vi "MasterAquisitionFile_2P_V2.vi"() -> ()   [LabVIEW 2020]
uses:
  <vilib>/userDefined/High Color/IMAQdx.ctl
  <vilib>/vision/driver/IMAQdx.llb/IMAQdx Camera Control Mode.ctl
  <vilib>/vision/driver/IMAQdx.llb/IMAQdx Acquisition Mode.ctl
  <vilib>/vision/driver/IMAQdx.llb/IMAQdx Buffer Number Mode.ctl
  <vilib>/DAQmx/write.llb/DAQmx Write (Digital 1D Wfm NChan NSamp).vi
  <vilib>/DAQmx/read.llb/DAQmx Read (Digital 1D Bool 1Chan 1Samp).vi
  <vilib>/DAQmx/read.llb/DAQmx Read (Analog 1D Wfm NChan NSamp).vi
  <vilib>/Waveform/DWDTOps.llb/DWDT Digital to Boolean Array.vi
  <vilib>/DAQmx/create/channels.llb/DAQmx Create Channel (DO-Digital Output).vi
  <vilib>/DAQmx/configure/timing.llb/DAQmx Timing (Sample Clock).vi
  <vilib>/Waveform/DWDTOps.llb/DWDT Uncompress Digital.vi
  <vilib>/DAQmx/miscellaneous.llb/DAQmx Fill In Error Info.vi
  <vilib>/DAQmx/create/channels.llb/DAQmx Create Channel (DI-Digital Input).vi
  <vilib>/DAQmx/create/channels.llb/DAQmx Create Channel (AI-Voltage-Basic).vi
  <vilib>/DAQmx/configure/trigger.llb/DAQmx Start Trigger (Digital Edge).vi
  <vilib>/DAQmx/create/channels.llb/DAQmx Create Channel (CO-Pulse Generation-Frequency).vi
  <vilib>/DAQmx/configure/timing.llb/DAQmx Timing (Implicit).vi
  <vilib>/vision/driver/NI_Vision_Acquisition_Software.lvlib
  <resource>/objmgr/imaqdx.rc
  <resource>/objmgr/daqmx.rc
panel:
  out "Auditory":bool
  out "RPad":bool
  out "LPad":bool
  in  "Sol Stim Parameters":cluster{"Fs":dbl, "Samples":dbl}
  in  "LED Stim Parameters":cluster{"Fs":dbl, "Samples":dbl}
  in  "Generate Stimuli":bool=TRUE
  in  "Sol Duty Cycle (%)":dbl=10.0
  in  "Sol Freq":dbl=1.0
  in  "Sol Dur (s)":dbl=1.0
  in  "LED Duty Cycle (%)":dbl=10.0
  in  "LED Freq":dbl=10.0
  in  "LED Dur (s)":dbl=2.0
  out "Stimulus Order":digitalwaveform[](graph)=[{"t0"=timestamp(0 s since 1904-01-01), "dt"=5e-05, "Y"={"transitions"=[], "data"=array18000000x1[18000000 elements]}}, {"t0"=timestamp(0 s since 1904-01-01), "dt"=5e-05, "Y"={"transitions"=[], "data"=array18000000x1[18000000 elements]}}, {"t0"=timestamp(0 s since 1904-01-01), "dt"=5e-05, "Y"={"transitions"=[], "data"=array18000000x1[18000000 elements]}}, {"t0"=timestamp(0 s since 1904-01-01), "dt"=5e-05, "Y"={"transitions"=[], "data"=array18000000x1[18000000 elements]}}]
  out "Solenoid Stim":digitalwaveform(graph)={"t0"=timestamp(0 s since 1904-01-01), "dt"=5e-05, "Y"={"transitions"=[], "data"=array20000x1[20000 elements]}}
  in  "Trial Offset (s)":dbl=15.0
  in  "Interstim (s)":dbl=30.0
  in  "Right Pad":dbl=1.0
  in  "Left Pad":dbl=1.0
  in  "Auditory":dbl=1.0
  in  "LED":dbl
  out "?":T1(plugin-control)
  out "Web Cam Fs 2":dbl(knob) scale=0.0..200.0
  out "MScan Cam":bool
  out "?":T1(plugin-control)
  in  "stop":bool
  out "?":T1(plugin-control)
  out "Web Cam Fs":dbl(knob) scale=0.0..200.0
  out "Behav Cam":bool
  out "Complete":bool
  out "Whisk Cam":bool
  out "Analog":bool
  out "MScan Trig":bool
  out "?":bool[](array[boolean])=[TRUE]
  out "Hexadecimal Data":u32=1 format="%x"
  out "Time Elapsed (Min)":cluster{dbl, dbl}(slide)={16.0, 0.028422350000000002} scale=0.0..16.0 scale format="%#_2g"
  out "Whisker Camera":bool
  out "Analog Data":bool
  out "Analog Samples":i32
  in  "Analog Channel\n Labels":string[](array[string])=["forceSensor", "AudSol", "LPadSol", "RPadSol", "", "", "", ""]
  in  "?":cluster{"Analog Fs":u16}={"Analog Fs"=20000} {"Analog Fs" format="%0.0f"}
  in  "?":cluster{"WhiskerCam Fs":u16}={"WhiskerCam Fs"=150}
  out "Notes Size":i32=7
  out "Notes Reversed":string[](array[string])=["Experimenter", "Animal ID", "Isoflurane time", "Amplifier Gain", "Session ID", "Hemisphere", "Solenoid PSI"]
  out "Notes Array":string[](array[string])=["Solenoid PSI", "Hemisphere", "Session ID", "Amplifier Gain", "Isoflurane time", "Animal ID", "Experimenter"]
  in  "Notes:":T2={"Experimenter"="Kevin\n", "Animal ID"="T201", "Isoflurane time"="1110", "Amplifier Gain"="10000", "Session ID"="Imaging Session Three", "Hemisphere"="RH", "Solenoid PSI"="10"}
  in  "Target Path":path=path "C:/Users/klt8/Documents/T201/Imaging Session 3 - 7 Apr. 2021" caption="Final Saved File Location"
  out "Dropped":u32(slide) caption="Whisk Cam" scale=0.0..150.0
  out "Current File Name":string="190611_17_21_53"
  in  "Time (min)":dbl(knob)=16.0 min=0.5 max=20.0 step=0.5 scale=0.0..20.0 scale format="%#_3g"
  in  "Temp Path":path=path "C:/Users/klt8/Documents/LabVIEW Temp Files" caption="Temporary File Path"
  out "Last Whisk Buffer":u32=251
  out "Whisk Cam Fs":dbl(knob) scale=0.0..200.0 scale format="%#1_6g"
  # "Notes"
  # "Dropped Frames"
  # "LPAD"
  # "RPAD"
  # "AUD"
  # "AnalogFs"
  # "WhiskFs"
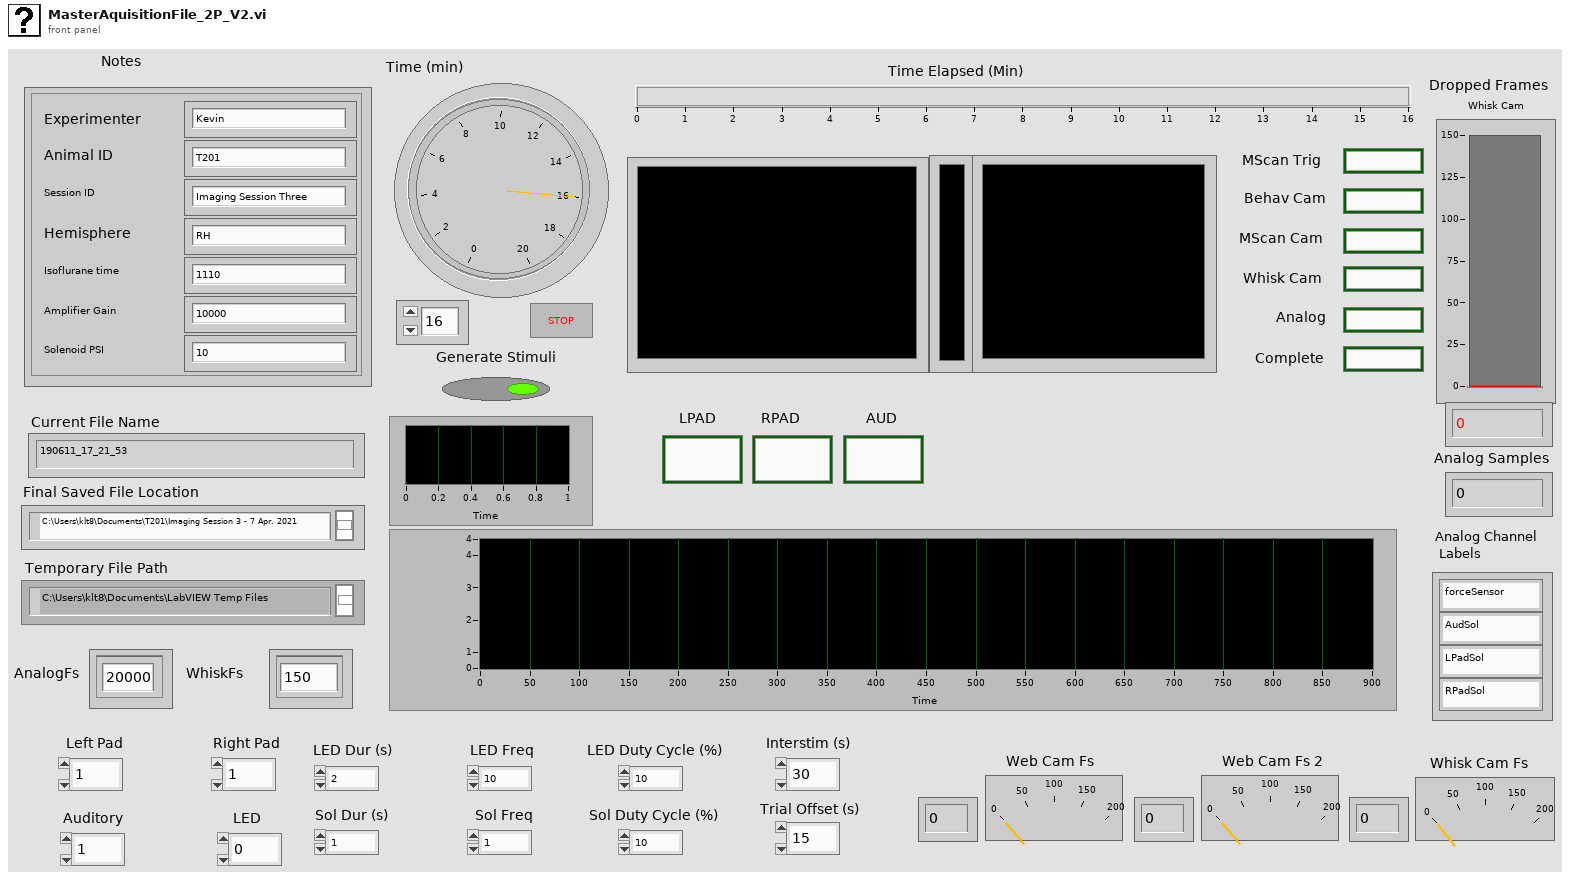
[diagram p1: front panel]
types:
  T1 = typedef "IMAQ Image.ctl" = refnum<image>
  T2 = cluster{"Experimenter":string, "Animal ID":string, "Isoflurane time":string, "Amplifier Gain":string, "Session ID":string, "Hemisphere":string, "Solenoid PSI":string}
  T3 = typedef "IMAQdx.ctl" = refnum<k21>
  T4 = typedef "NI_Vision_Acquisition_Software.lvlib/IMAQdx Camera Control Mode.ctl" = enum32{"Controller", "Listener"}
  T5 = enum16{"open", "open or create", "create or replace", "create", "open (read-only)"}
  T6 = enum16{"open", "replace", "create", "open or create", "replace or create", "replace or create with confirmation"}
  T7 = typedef "NI_Vision_Acquisition_Software.lvlib/IMAQdx Acquisition Mode.ctl" = enum32{"One Shot", "Continuous"}
  T8 = enum16{"big-endian, network order", "native, host order", "little-endian"}
  T9 = typedef "NI_Vision_Acquisition_Software.lvlib/IMAQdx Buffer Number Mode.ctl" = enum32{"Next", "Last", "Buffer Number", "Every", "Last New"}
  T10 = typedef "Image Type" = u32
  T11 = typedef "IMAQ AVI2 Refnum.ctl" = refnum<k20>
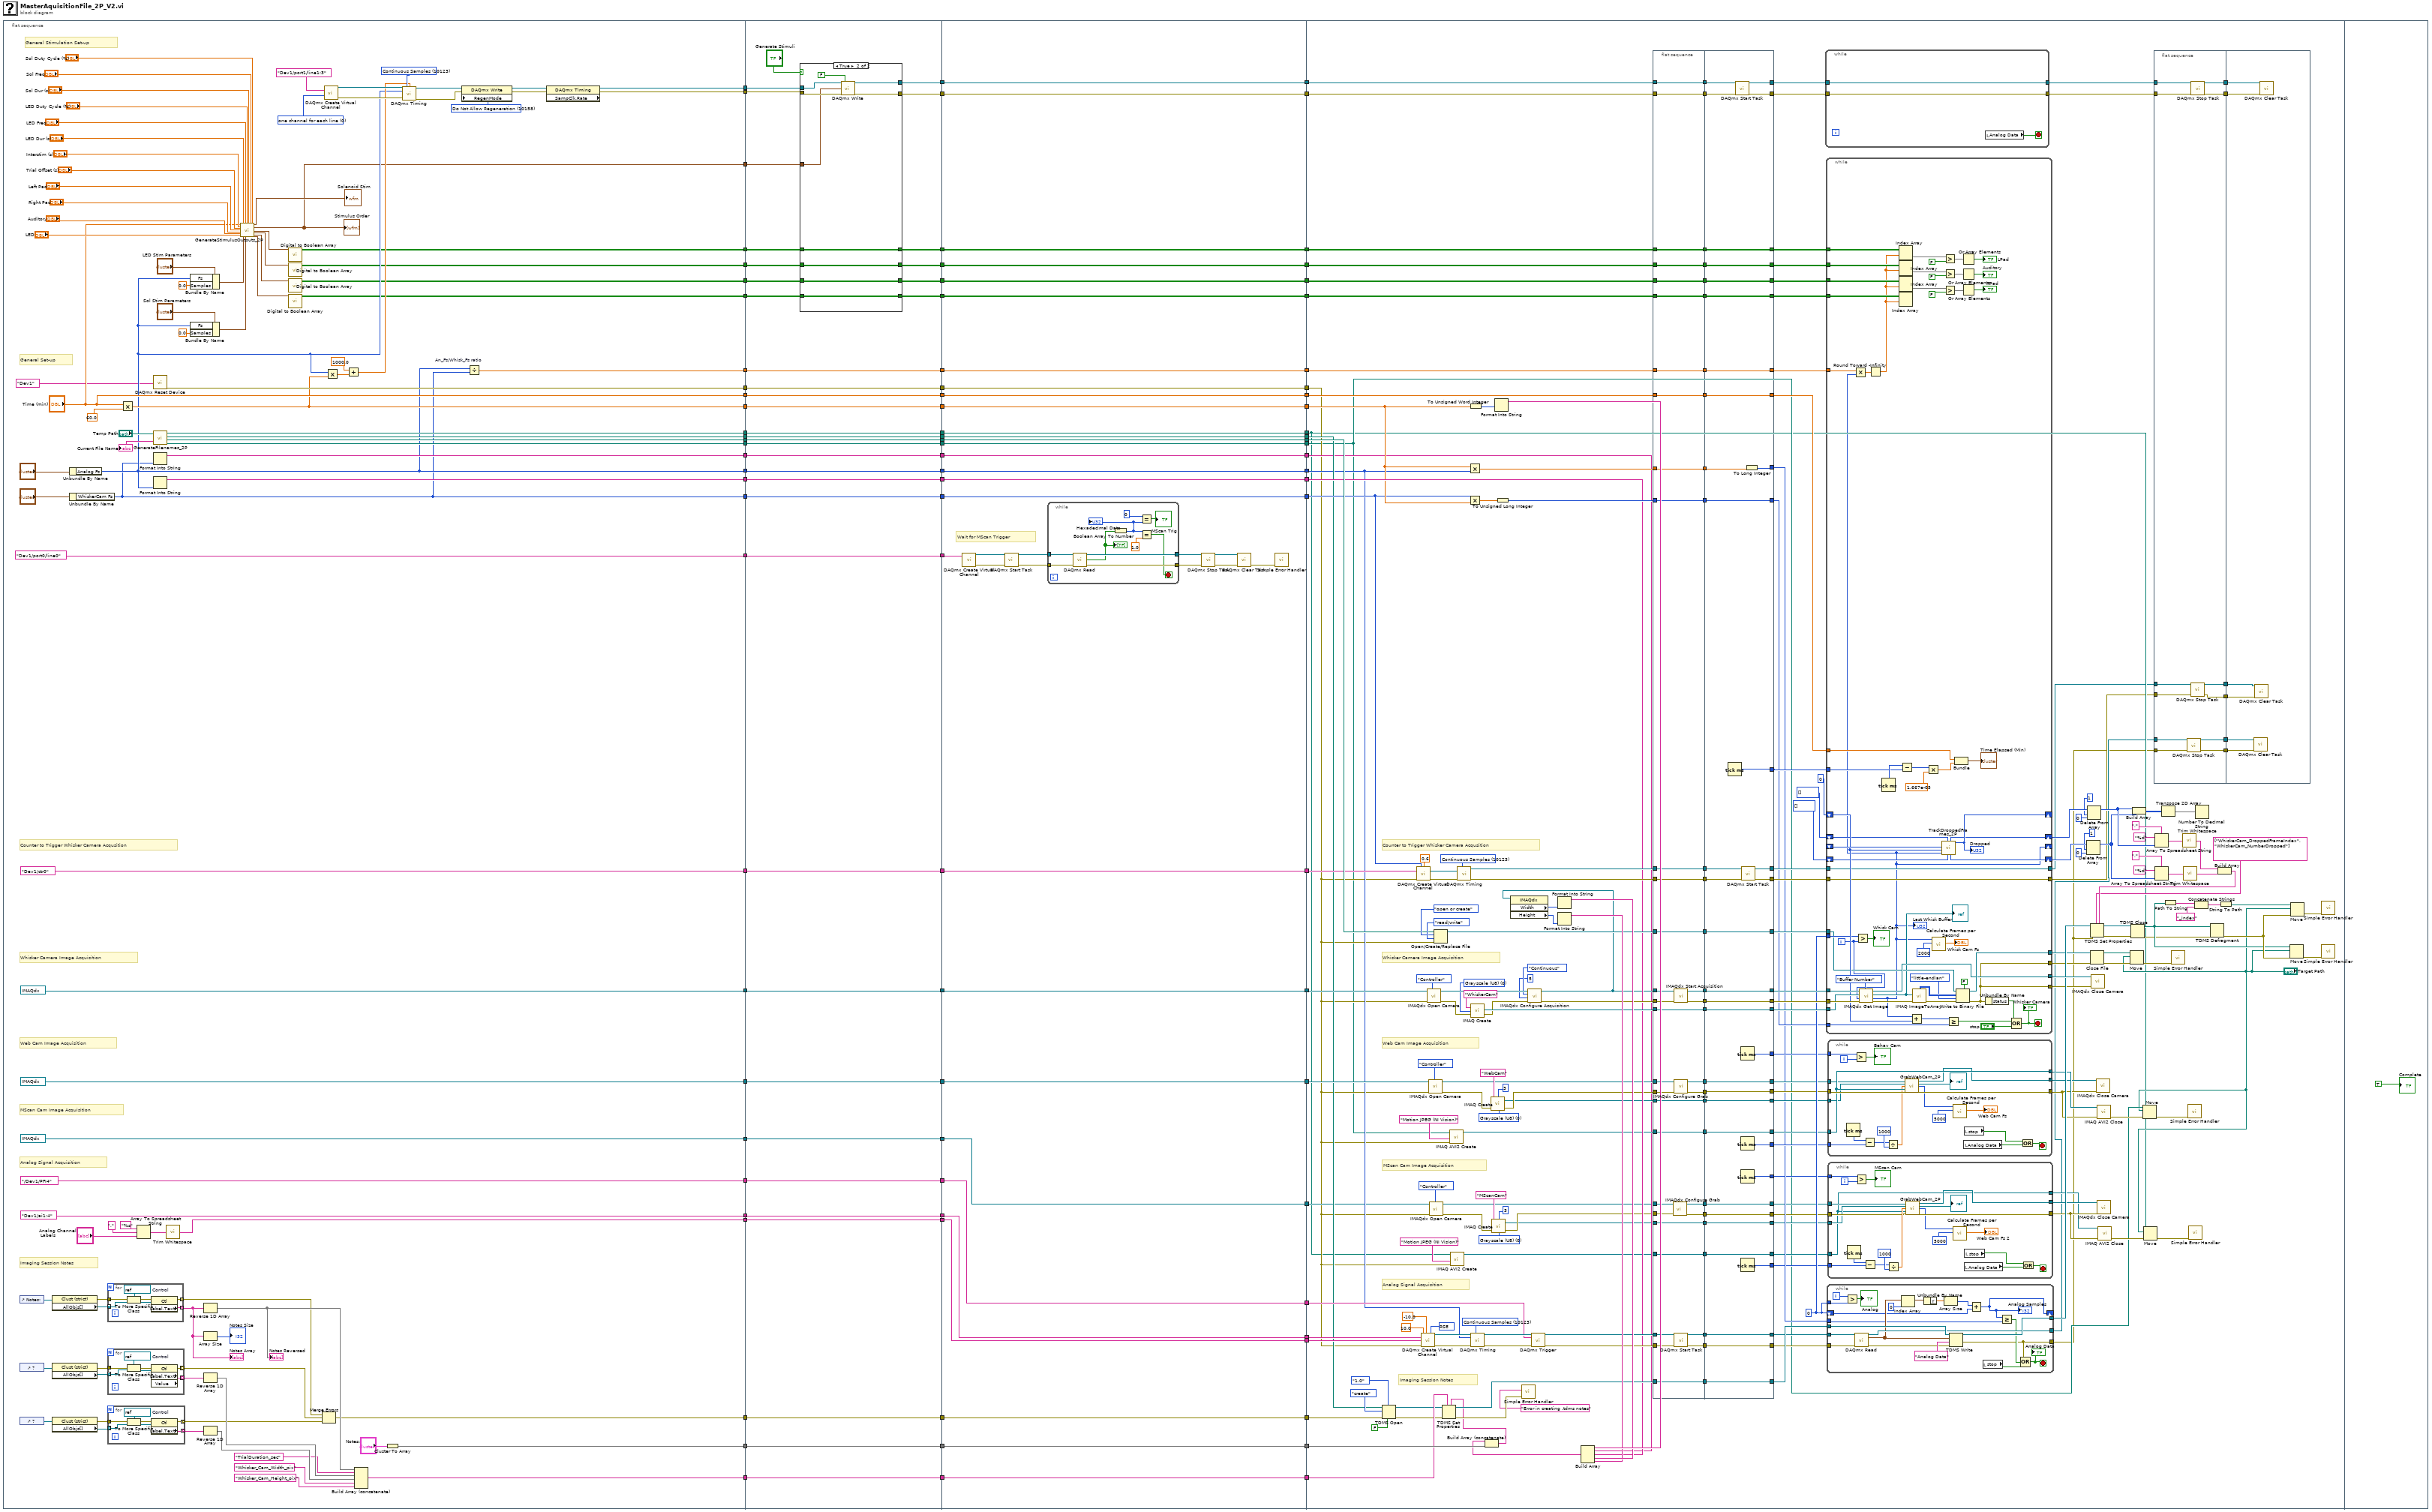
[diagram p0: block diagram]
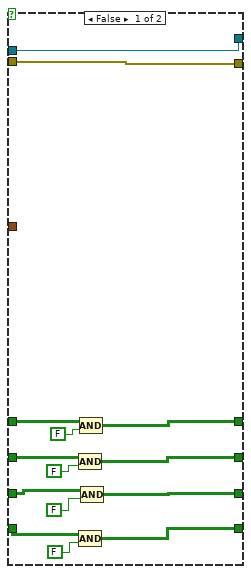
[diagram p2: hidden frame]
diagram:
  n1 = flat-sequence {
    tunnel: [tag "/Dev1/PFI4" ("Whisk Cam Trigger")] -> w59
    tunnel: [w109] -> w57
    tunnel: ["Time (min)"] -> w55
    tunnel: [w156] -> w53
    tunnel: [w155] -> w51
    tunnel: [w107] -> w49
    tunnel: [w106] -> w47
    tunnel: [w154] -> w45
    tunnel: [tag "Dev1/ctr0" ("Whisk Cam Counter")] -> w43
    tunnel: [w153] -> w41
    tunnel: [tag "Dev1/ai1:4" ("Analog Input Channels")] -> w39
    tunnel: [T3 "cam1" ("Whisker Cam ID")] -> w37
    tunnel: [w152] -> w35
    tunnel: [w150] -> w33
    tunnel: [w151] -> w31
    tunnel: [T3 "cam2" ("WebCam ID")] -> w29
    tunnel: [tag "Dev1/port0/line0" ("MScan Trigger")] -> w27
    tunnel: [w147] -> w25
    tunnel: [w146] -> w23
    tunnel: [w145] -> w21
    tunnel: [T3 "cam7" ("WebCam ID 2")] -> w19
    tunnel: [w144] -> w17
    tunnel: [w105] -> w9
    tunnel: [w94] -> w7
    tunnel: [w93] -> w6
    tunnel: [w92] -> w5
    tunnel: [w91] -> w4
    tunnel: [w90] -> w3
    tunnel: [w89] -> w2
    tunnel: [w88] -> w1
    tunnel: w59 -> [w244]
    tunnel: [w244] -> w58
    tunnel: w57 -> [w243]
    tunnel: [w243] -> w56
    tunnel: w55 -> [w242]
    tunnel: [w242] -> w54
    tunnel: w53 -> [w241]
    tunnel: [w241] -> w52
    tunnel: w51 -> [w240]
    tunnel: [w240] -> w50
    tunnel: w49 -> [w239]
    tunnel: [w239] -> w48
    tunnel: w47 -> [w238]
    tunnel: [w238] -> w46
    tunnel: w45 -> [w237]
    tunnel: [w237] -> w44
    tunnel: w43 -> [w236]
    tunnel: [w236] -> w42
    tunnel: w41 -> [w235]
    tunnel: [w235] -> w40
    tunnel: w39 -> [w234]
    tunnel: [w234] -> w38
    tunnel: w37 -> [w233]
    tunnel: [w233] -> w36
    tunnel: w35 -> [w232]
    tunnel: [w232] -> w34
    tunnel: w33 -> [w231]
    tunnel: [w231] -> w32
    tunnel: w31 -> [w230]
    tunnel: [w230] -> w30
    tunnel: w29 -> [w229]
    tunnel: [w229] -> w28
    tunnel: w27 -> [w228]
    tunnel: [w228] -> w26
    tunnel: w25 -> [w227]
    tunnel: [w227] -> w24
    tunnel: w23 -> [w226]
    tunnel: [w226] -> w22
    tunnel: w21 -> [w225]
    tunnel: [w225] -> w20
    tunnel: w19 -> [w224]
    tunnel: [w224] -> w18
    tunnel: w17 -> [w223]
    tunnel: [w223] -> w16
    tunnel: [w214] -> w15
    tunnel: [w213] -> w14
    tunnel: [w212] -> w13
    tunnel: [w211] -> w12
    tunnel: [w210] -> w11
    tunnel: [w209] -> w10
    tunnel: w9 -> [w222]
    tunnel: [w222] -> w8
    tunnel: w7 -> [w221]
    tunnel: w6 -> [w220]
    tunnel: w5 -> [w219]
    tunnel: w4 -> [w218]
    tunnel: w3 -> [w217]
    tunnel: w2 -> [w216]
    tunnel: w1 -> [w215]
    tunnel: [w283] -> w87
    tunnel: [w295] -> w86
    tunnel: [w296] -> w85
    tunnel: [w297] -> w84
    tunnel: [w298] -> w83
    tunnel: [w285] -> w82
    tunnel: [w299] -> w81
    tunnel: [w284] -> w80
    tunnel: [w300] -> w79
    tunnel: [w301] -> w78
    tunnel: [w302] -> w77
    tunnel: [w303] -> w76
    tunnel: [w304] -> w75
    tunnel: [w305] -> w74
    tunnel: [w306] -> w73
    tunnel: w58 -> [w306]
    tunnel: w56 -> [w305]
    tunnel: w54 -> [w304]
    tunnel: w52 -> [w303]
    tunnel: w50 -> [w302]
    tunnel: w48 -> [w301]
    tunnel: w46 -> [w300]
    tunnel: w44 -> [w284]
    tunnel: w42 -> [w299]
    tunnel: w40 -> [w285]
    tunnel: w38 -> [w298]
    tunnel: w36 -> [w297]
    tunnel: w34 -> [w296]
    tunnel: w32 -> [w295]
    tunnel: w30 -> [w283]
    tunnel: [w281] -> w72
    tunnel: w28 -> [w281]
    tunnel: w26 -> [w282]
    tunnel: w24 -> [w280]
    tunnel: [w280] -> w71
    tunnel: w22 -> [w279]
    tunnel: w20 -> [w278]
    tunnel: [w279] -> w70
    tunnel: [w278] -> w69
    tunnel: w18 -> [w277]
    tunnel: [w277] -> w68
    tunnel: w16 -> [w276]
    tunnel: [w276] -> w67
    tunnel: [w275] -> w66
    tunnel: w15 -> [w275]
    tunnel: [w274] -> w65
    tunnel: w14 -> [w274]
    tunnel: [w273] -> w64
    tunnel: w13 -> [w273]
    tunnel: [w272] -> w63
    tunnel: w12 -> [w272]
    tunnel: [w271] -> w62
    tunnel: w11 -> [w271]
    tunnel: w10 -> [w270]
    tunnel: [w270] -> w61
    tunnel: [w269] -> w60
    tunnel: w8 -> [w269]
    tunnel: w87 -> [w429]
    tunnel: w86 -> [w439]
    tunnel: w85 -> [w373]
    tunnel: w84 -> [w438]
    tunnel: w83 -> [w437]
    tunnel: w82 -> [w436]
    tunnel: w81 -> [w435]
    tunnel: w80 -> [w434]
    tunnel: w79 -> [w398]
    tunnel: w78 -> [w388]
    tunnel: w77 -> [w433]
    tunnel: w76 -> [w387]
    tunnel: w75 -> [w426]
    tunnel: w74 -> [w432]
    tunnel: w73 -> [w431]
    tunnel: w72 -> [w417]
    tunnel: w71 -> [w352]
    tunnel: w70 -> [w394]
    tunnel: w69 -> [w392]
    tunnel: w68 -> [w375]
    tunnel: w67 -> [w350]
    tunnel: w66 -> [w320]
    tunnel: w65 -> [w318]
    tunnel: w64 -> [w324]
    tunnel: w63 -> [w323]
    tunnel: w62 -> [w322]
    tunnel: w61 -> [w321]
    tunnel: w60 -> [w340]
    frame #0 {
      w124 = 10158 items=["Allow Regeneration"=10097, "Do Not Allow Regeneration"=10158] ("RegenMode")
      w125 = 10123 items=["Finite Samples"=10178, "Continuous Samples"=10123, "Hardware Timed Single Point"=12522] ("sample mode")
      w128 = 0 items=["one channel for each line", "one channel for all lines"] ("line grouping")
      # "General Stimulation Set-up"
      # "MScan Cam Image Acquisition"
      # "General Set-up"
      # "Whisker Camera Image Acquisition"
      # "Imaging Session Notes"
      # "Counter to Trigger Whisker Camera Acqusition"
      # "Web Cam Image Acquisition"
      # "Analog Signal Acquisition"
      n2 = control-ref of="Notes:"() -> (w172:refnum<vi>)
      n3 = control-ref of="?"() -> (w170:refnum<vi>)
      n4 = control-ref of="?"() -> (w163:refnum<vi>)
      n5 = property class="Clust (strict)"(reference=w172) -> (error out=w171:errorcluster, "AllObjs[]"=w173:refnum<vi>[])  [unwired: 1 in, 1 out]
      n6 = property class="Clust (strict)"(reference=w170) -> (error out=w168:errorcluster, "AllObjs[]"=w169:refnum<vi>[])  [unwired: 1 in, 1 out]
      n7 = property class="Clust (strict)"(reference=w163) -> (error out=w164:errorcluster, "AllObjs[]"=w166:refnum<vi>[])  [unwired: 1 in, 1 out]
      n8 = Unbundle By Name("?") -> ("Analog Fs"=w107:u16)
      n9 = Unbundle By Name("?") -> ("WhiskerCam Fs"=w106:u16)
      n10 = for {
        tunnel: [w191] -> w178 mode=indexing
        tunnel: w173 -> [w190] mode=indexing
        tunnel: w171 -> [w189]
        tunnel: [w187] -> w177 mode=indexing
        w192 = refnum<vi> refnum  # Control
        n11 = To More Specific Class(target class=w192, reference=w190, error in=w189) -> (specific class reference=w193:refnum<vi>, error out=w188:errorcluster)
        n12 = property class="Ctl"(reference=w193, error in=w188) -> (error out=w187:errorcluster, "Label.Text"=w191:string)  [unwired: 1 out]
      }
      "Notes Array" <- w178
      n13 = for {
        tunnel: [w198] -> w167 mode=indexing
        tunnel: w169 -> [w197] mode=indexing
        tunnel: w168 -> [w196]
        tunnel: [w194] -> w176 mode=indexing
        w199 = refnum<vi> refnum  # Control
        n14 = To More Specific Class(target class=w199, reference=w197, error in=w196) -> (specific class reference=w200:refnum<vi>, error out=w195:errorcluster)
        n15 = property class="Ctl" props=["Label", "Text", "Value"](reference=w200, error in=w195) -> (error out=w194:errorcluster, "Label.Text"=w198:string)  [unwired: 2 out]
      }
      n16 = for {
        tunnel: [w205] -> w165 mode=indexing
        tunnel: w166 -> [w204] mode=indexing
        tunnel: w164 -> [w203]
        tunnel: [w201] -> w175 mode=indexing
        w206 = refnum<vi> refnum  # Control
        n17 = To More Specific Class(target class=w206, reference=w204, error in=w203) -> (specific class reference=w207:refnum<vi>, error out=w202:errorcluster)
        n18 = property class="Ctl"(reference=w207, error in=w202) -> (error out=w201:errorcluster, "Label.Text"=w205:string)  [unwired: 1 out]
      }
      n19 = Multiply(x="Time (min)", y=60.0) -> (x*y=w109:dbl)
      n20 = Array To Spreadsheet String(delimiter (Tab)=",", array="Analog Channel\n Labels", 3:"%s" ("format string")) -> (spreadsheet string=w180:string)
      n21 = call <vilib>:"DAQmx Reset Device.vi"("device in"=tag "Dev1" ("NI Board")) -> ("error out"=w152:errorcluster)  [unwired: 14 in]
      n22 = call "GenerateFilenames_2P.vi"("path"="Temp Path") -> ("WebCam Path"=w147:path, "Basler Path"=w150:path, "TDMS Path"=w145:path, "MScan Path"=w144:path, "Analog file name"=→"Current File Name":string)  [unwired: 2 in]
      n23 = Format Into String(w106) -> (resulting string=w156:string)  [unwired: 3 in, 1 out]
      n24 = Format Into String(w107) -> (resulting string=w155:string)  [unwired: 3 in, 1 out]
      n25 = call <vilib>:"Trim Whitespace.vi"("string"=w180) -> ("trimmed string"=w153:string)  [unwired: 1 in]
      n26 = Bundle By Name(cluster="LED Stim Parameters", "Fs"=w107, "Samples"=0.0) -> (w114:cluster{"Fs":dbl, "Samples":dbl})
      n27 = Bundle By Name(cluster="Sol Stim Parameters", "Fs"=w107, "Samples"=0.0) -> (w113:cluster{"Fs":dbl, "Samples":dbl})
      n28 = Reverse 1D Array(array=w178) -> (reversed array=w179:string[])
      "Notes Reversed" <- w179
      n29 = Array Size(array=w178) -> (size(s)=→"Notes Size":i32)
      n30 = Reverse 1D Array(array=w167) -> (reversed array=w185:string[])
      n31 = Reverse 1D Array(array=w165) -> (reversed array=w186:string[])
      n32 = call "GenerateStimulusOutputs_2P.vi"("Trial duration (min)"="Time (min)", "Rest duration(s)"="Interstim (s)", "trial offset (s)"="Trial Offset (s)", "Left Pad"="Left Pad", "Right Pad"="Right Pad", "Auditory"="Auditory", "LED"="LED", "LED Stim Duration (s)"="LED Dur (s)", "LED Stim Parameters"=w114, "LED Frequency"="LED Freq", "Sol Stim Parameters"=w113, "LED duty cycle (%)"="LED Duty Cycle (%)", "Sol Stim Duration (s)"="Sol Dur (s)", "Sol Frequency"="Sol Freq", "Sol Duty Cycle (%)"="Sol Duty Cycle (%)") -> ("Solenoid Stim Waveforms"=→"Solenoid Stim":digitalwaveform, "Stimulus Digital Outputs"=w90:digitalwaveform[], "Left Pad Out"=w103:digitalwaveform, "Auditory Out"=w130:digitalwaveform, "Right Pad Out"=w129:digitalwaveform, "LED Out"=w108:digitalwaveform)  [unwired: 7 in]
      "Stimulus Order" <- w90
      n33 = call-poly <vilib>:"Digital to Boolean Array.vi"("digital waveform"=w103) -> ("boolean array"=w89:bool[][])  [unwired: 9 in, 1 out]
      n34 = call-poly <vilib>:"Digital to Boolean Array.vi"("digital waveform"=w130) -> ("boolean array"=w92:bool[][])  [unwired: 9 in, 1 out]
      n35 = call-poly <vilib>:"Digital to Boolean Array.vi"("digital waveform"=w129) -> ("boolean array"=w91:bool[][])  [unwired: 9 in, 1 out]
      n36 = call-poly <vilib>:"Digital to Boolean Array.vi"("digital waveform"=w108) -> ("boolean array"=w88:bool[][])  [unwired: 9 in, 1 out]
      n37 = Merge Errors(w177, w176, w175) -> (w146:errorcluster)
      n38 = call-poly <vilib>:"DAQmx Create Virtual Channel.vi"("lines"=tag "Dev1/port1/line1:3", "line grouping"=w128) -> ("task out"=w127:refnum<k21>, "error out"=w126:errorcluster)  [unwired: 12 in]
      n39 = Multiply(x=w107, y=w109) -> (x*y=w112:dbl)
      n40 = Add(x=1000.0, y=w112) -> (x+y=w110:dbl)
      n41 = Build Array (concatenate)(w179, "TrialDuration_sec", w185, w186, "Whisker_Cam_Width_pix", "Whisker_Cam_Height_pix") -> (w151:string[])
      n42 = Cluster To Array(cluster="Notes:") -> (array=w154:string[])
      n43 = call-poly <vilib>:"DAQmx Timing.vi"("task/channels in"=w127, "sample mode"=w125, "samples per channel"=w110, "rate"=w107, "error in"=w126) -> ("task out"=w121:refnum<k21>, "error out"=w120:errorcluster)  [unwired: 9 in]
      n44 = property class="DAQmx Write"(reference=w121, error in=w120, "RegenMode"=w124) -> (reference out=w122:refnum<k21>, error out=w123:errorcluster)
      n45 = Divide "An_Fs/Whisk_Fs ratio"(x=w107, y=w106) -> (x/y=w105:dbl)
      n46 = property class="DAQmx Timing" props=["SampClk.Rate"](reference=w122, error in=w123) -> (reference out=w94:refnum<k21>, error out=w93:errorcluster)  [unwired: 1 out]
    }
    frame #1 {
      n47 = case shown="True" "Generate Stimuli" {
        tunnel: w221 -> [w258 w268]
        tunnel: w220 -> [w257 w267]
        tunnel: [w258 w266] -> w214
        tunnel: [w257 w265] -> w213
        tunnel: w219 -> [w253 w264]
        tunnel: w218 -> [w254 w263]
        tunnel: [w247 w261] -> w212
        tunnel: [w256 w264] -> w211
        tunnel: [w255 w263] -> w210
        tunnel: [w246 w260] -> w209
        tunnel: w217 -> [_ w262]
        tunnel: w216 -> [w248 w261]
        tunnel: w215 -> [w245 w260]
        frame False {
          n48 = Compound Arithmetic op=AND(w253, FALSE) -> (w256:bool[][])
          n49 = Compound Arithmetic op=AND(w245, FALSE) -> (w246:bool[][])
          n50 = Compound Arithmetic op=AND(w248, FALSE) -> (w247:bool[][])
          n51 = Compound Arithmetic op=AND(w254, FALSE) -> (w255:bool[][])
        }
        frame True {
          n52 = call-poly <vilib>:"DAQmx Write.vi"("task/channels in"=w268, "auto start"=FALSE, "data"=w262, "error in"=w267) -> ("task out"=w266:refnum<k21>, "error out"=w265:errorcluster)  [unwired: 9 in, 1 out]
        }
      }
    }
    frame #2 {
      # "Wait for MScan Trigger"
      n53 = call-poly <vilib>:"DAQmx Create Virtual Channel.vi"("lines"=w282) -> ("task out"=w290:refnum<k21>, "error out"=w291:errorcluster)  [unwired: 13 in]
      n54 = call <vilib>:"DAQmx Start Task.vi"("task/channels in"=w290, "error in"=w291) -> ("task out"=w294:refnum<k21>, "error out"=w293:errorcluster)  [unwired: 12 in]
      n55 = while {
        tunnel: w294 -> [w316]
        tunnel: w293 -> [w315]
        tunnel: [w313] -> w288
        tunnel: [w314] -> w289
        stop <- w308 stop-if-true
        n56 = call-poly <vilib>:"DAQmx Read.vi"("task/channels in"=w316, "error in"=w315) -> ("task out"=w314:refnum<k21>, "data"=w312:bool[], "error out"=w313:errorcluster)  [unwired: 11 in]
        "?" <- w312
        n57 = Boolean Array To Number(Boolean array=w312) -> (number=w307:u32)
        "Hexadecimal Data" <- w307
        n58 = Equal?(x=w307, y=u32 0) -> (x = y?=→"MScan Trig":bool)
        n59 = Equal?(x=w307, y=1.0) -> (x = y?=w308:bool)
      }
      n60 = call <vilib>:"DAQmx Stop Task.vi"("task/channels in"=w289, "error in"=w288) -> ("task out"=w287:refnum<k21>, "error out"=w286:errorcluster)  [unwired: 12 in]
      n61 = call <vilib>:"DAQmx Clear Task.vi"("task in"=w287, "error in"=w286) -> ("error out"=w292:errorcluster)  [unwired: 13 in]
      n62 = call <vilib>:"Simple Error Handler.vi"("error in (no error)"=w292) -> ()  [unwired: 4 in, 5 out]
    }
    frame #3 {
      w378 = T10 0 items=["Grayscale (U8)", "Grayscale (I16)", "Grayscale (SGL)", "Complex (CSG)", "RGB (U32)", "HSL (U32)", "RGB (U64)", "Grayscale (U16)"] ("Image Type")
      w421 = T10 0 items=["Grayscale (U8)", "Grayscale (I16)", "Grayscale (SGL)", "Complex (CSG)", "RGB (U32)", "HSL (U32)", "RGB (U64)", "Grayscale (U16)"] ("Image Type")
      w405 = u32 0 ("y")
      w448 = 10123 items=["Finite Samples"=10178, "Continuous Samples"=10123, "Hardware Timed Single Point"=12522] ("sample mode")
      w447 = 10083 items=["default"=-1, "RSE"=10083, "NRSE"=10078, "Differential"=10106, "Pseudodifferential"=12529] ("input terminal configuration")
      w449 = 10123 items=["Finite Samples"=10178, "Continuous Samples"=10123, "Hardware Timed Single Point"=12522] ("sample mode")
      w445 = T10 0 items=["Grayscale (U8)", "Grayscale (I16)", "Grayscale (SGL)", "Complex (CSG)", "RGB (U32)", "HSL (U32)", "RGB (U64)", "Grayscale (U16)"] ("Image Type")
      # "MScan Cam Image Acquisition"
      # "Whisker Camera Image Acquisition"
      # "Imaging Session Notes"
      # "Counter to Trigger Whisker Camera Acqusition"
      # "Web Cam Image Acquisition"
      # "Analog Signal Acquisition"
      n63 = TDMS Open(6:FALSE ("disable buffering? (T)"), 7:enum16{"1.0", "2.0"}."1.0" ("file format version (2.0)"), 8:w394, 10:T5."create" ("operation (0:open)"), 11:w392) -> (0:w391:errorcluster, 3:w390:refnum<k34>)  [unwired: 2 in]
      n64 = call-poly <vilib>:"DAQmx Create Virtual Channel.vi"("frequency"=w398, "duty cycle"=0.6, "counter"=w435, "error in"=w373) -> ("task out"=w472:refnum<k21>, "error out"=w473:errorcluster)  [unwired: 10 in]
      n65 = call-poly <vilib>:"DAQmx Create Virtual Channel.vi"("maximum value"=10.0, "minimum value"=-10.0, "input terminal configuration"=w447, "physical channels"=w437, "name to assign"=w436, "error in"=w373) -> ("task out"=w481:refnum<k21>, "error out"=w482:errorcluster)  [unwired: 8 in]
      n66 = call <vilib>:"IMAQdx Open Camera.vi"("Camera Control Mode"=IMAQdx_Camera_Control_Mode."Controller", "error in"=w373, "Session In"=w438) -> ("error out"=w470:errorcluster, "Session Out"=w469:T3)  [unwired: 7 in]
      n67 = call <vilib>:"IMAQdx Open Camera.vi"("Camera Control Mode"=IMAQdx_Camera_Control_Mode."Controller", "error in"=w373, "Session In"=w417) -> ("error out"=w418:errorcluster, "Session Out"=w416:T3)  [unwired: 7 in]
      n68 = call <vilib>:"IMAQdx Open Camera.vi"("Camera Control Mode"=IMAQdx_Camera_Control_Mode."Controller", "error in"=w373, "Session In"=w375) -> ("error out"=w376:errorcluster, "Session Out"=w370:T3)  [unwired: 7 in]
      n69 = Open/Create/Replace File(file path (use dialog)=w439, error in=w373, operation (0:open)=T6."open or create", access (0:read/write)=enum16{"read/write", "read-only", "write-only"}."read/write") -> (refnum out=w480:refnum<file>)  [unwired: 2 in, 2 out]
      n70 = call "IMAQ AVI2 Create"("error in (no error)"=w373, "Codec"="Motion JPEG (NI Vision)", "AVI Path"=w352) -> ("AVI Refnum"=w400:T11)  [unwired: 7 in, 1 out]
      n71 = call "IMAQ AVI2 Create"("error in (no error)"=w373, "Codec"="Motion JPEG (NI Vision)", "AVI Path"=w350) -> ("AVI Refnum"=w366:T11)  [unwired: 7 in, 1 out]
      n72 = call-poly <vilib>:"DAQmx Timing.vi"("task/channels in"=w472, "sample mode"=w449, "error in"=w473) -> ("task out"=w490:refnum<k21>, "error out"=w491:errorcluster)  [unwired: 11 in]
      n73 = Multiply(x=w432, y=w388) -> (x*y=w518:dbl)
      n74 = Multiply(x=w398, y=w432) -> (x*y=w519:dbl)
      n75 = To Unsigned Word Integer(number=w432) -> (unsigned 16bit integer=w505:u16)
      n76 = call "IMAQ Create"("Image Name"="WhiskerCam", "Image Type"=w445, "error in (no error)"=w470) -> ("New Image"=w508:T1, "error out"=w471:errorcluster)  [unwired: 2 in]
      n77 = call-poly <vilib>:"DAQmx Timing.vi"("task/channels in"=w481, "sample mode"=w448, "rate"=w388, "error in"=w482) -> ("task out"=w483:refnum<k21>, "error out"=w484:errorcluster)  [unwired: 10 in]
      n78 = call "IMAQ Create"("Border Size"=3, "Image Name"="WebCam", "Image Type"=w421, "error in (no error)"=w418) -> ("New Image"=w414:T1, "error out"=w415:errorcluster)  [unwired: 1 in]
      n79 = call "IMAQ Create"("Border Size"=3, "Image Name"="MScanCam", "Image Type"=w378, "error in (no error)"=w376) -> ("New Image"=w360:T1, "error out"=w371:errorcluster)  [unwired: 1 in]
      n80 = Format Into String(w505) -> (resulting string=w527:string)  [unwired: 3 in, 1 out]
      n81 = To Unsigned Long Integer(number=w519) -> (unsigned 32bit integer=w520:u32)
      n82 = call <vilib>:"IMAQdx Configure Acquisition.vi"("error in"=w471, "Number of Buffers"=u32 5, "Continuous?"=IMAQdx_Acquisition_Mode."Continuous", "Session In"=w469) -> ("error out"=w475:errorcluster, "Session Out"=w389:T3)  [unwired: 6 in]
      n83 = property class="IMAQdx"(reference=w389) -> ("Width"=w506:u32, "Height"=w507:u32)  [unwired: 1 in, 2 out]
      n84 = call-poly <vilib>:"DAQmx Trigger.vi"("task/channels in"=w483, "source"=w431, "error in"=w484) -> ("task out"=w485:refnum<k21>, "error out"=w486:errorcluster)  [unwired: 11 in]
      n85 = Format Into String(w506) -> (resulting string=w526:string)  [unwired: 3 in, 1 out]
      n86 = Format Into String(w507) -> (resulting string=w525:string)  [unwired: 3 in, 1 out]
      n87 = Build Array(w527, w387, w433, w526, w525) -> (w385:string[])
      n88 = Build Array (concatenate)(w434, w385) -> (w440:string[])
      n89 = TDMS Set Properties(5:w440, 7:w429, 8:w391, 11:w390) -> (0:w504:errorcluster, 3:w503:refnum<k34>)  [unwired: 2 in, 2 out]
      n90 = call <vilib>:"Simple Error Handler.vi"("error source (\" \")"="Error in creating .tdms notes" ("error source (\" \")"), "error in (no error)"=w504) -> ()  [unwired: 3 in, 5 out]
      n91 = flat-sequence {
        tunnel: w389 -> [w658]
        tunnel: w475 -> [w657]
        tunnel: [w656] -> w538
        tunnel: [w655] -> w537
        tunnel: [w654] -> w536
        tunnel: w508 -> [w654]
        tunnel: [w653] -> w535
        tunnel: w480 -> [w653]
        tunnel: w485 -> [w652]
        tunnel: w486 -> [w651]
        tunnel: [w650] -> w534
        tunnel: [w649] -> w533
        tunnel: [w648] -> w532
        tunnel: w503 -> [w648]
        tunnel: w490 -> [w647]
        tunnel: [w647] -> w531
        tunnel: w491 -> [w646]
        tunnel: [w646] -> w530
        tunnel: w518 -> [w645]
        tunnel: [w645] -> w529
        tunnel: w520 -> [w644]
        tunnel: [w644] -> w528
        tunnel: w426 -> [w643]
        tunnel: [w643] -> w425
        tunnel: w416 -> [w642]
        tunnel: w415 -> [w641]
        tunnel: w414 -> [w640]
        tunnel: [w640] -> w413
        tunnel: [w639] -> w412
        tunnel: [w638] -> w411
        tunnel: [w637] -> w401
        tunnel: w400 -> [w637]
        tunnel: w371 -> [w633]
        tunnel: w370 -> [w636]
        tunnel: [w635] -> w369
        tunnel: [w634] -> w368
        tunnel: [w632] -> w367
        tunnel: w366 -> [w632]
        tunnel: [w631] -> w361
        tunnel: w360 -> [w631]
        tunnel: [w630] -> w349
        tunnel: w324 -> [w630]
        tunnel: [w629] -> w348
        tunnel: w323 -> [w629]
        tunnel: [w628] -> w347
        tunnel: w322 -> [w628]
        tunnel: [w627] -> w346
        tunnel: w321 -> [w627]
        tunnel: [w626] -> w341
        tunnel: w340 -> [w626]
        tunnel: w320 -> [w624]
        tunnel: [w625] -> w319
        tunnel: w318 -> [w625]
        tunnel: [w624] -> w317
        tunnel: [w688] -> w427
        tunnel: [w687] -> w428
        tunnel: [w695] -> w476
        tunnel: w538 -> [w695]
        tunnel: [w694] -> w477
        tunnel: w537 -> [w694]
        tunnel: [w693] -> w478
        tunnel: w536 -> [w693]
        tunnel: [w692] -> w479
        tunnel: w535 -> [w692]
        tunnel: [w691] -> w488
        tunnel: w534 -> [w691]
        tunnel: [w690] -> w487
        tunnel: w533 -> [w690]
        tunnel: [w689] -> w489
        tunnel: w532 -> [w689]
        tunnel: w531 -> [w684]
        tunnel: w530 -> [w686]
        tunnel: w529 -> [w675]
        tunnel: w528 -> [w685]
        tunnel: [w685] -> w384
        tunnel: [w683] -> w468
        tunnel: w425 -> [w682]
        tunnel: [w682] -> w424
        tunnel: [w681] -> w404
        tunnel: w413 -> [w681]
        tunnel: [w680] -> w402
        tunnel: w412 -> [w680]
        tunnel: [w679] -> w403
        tunnel: w411 -> [w679]
        tunnel: [w678] -> w397
        tunnel: w401 -> [w677]
        tunnel: [w677] -> w399
        tunnel: [w676] -> w396
        tunnel: [w674] -> w383
        tunnel: [w673] -> w363
        tunnel: w369 -> [w673]
        tunnel: [w672] -> w362
        tunnel: w368 -> [w672]
        tunnel: [w671] -> w353
        tunnel: w367 -> [w671]
        tunnel: [w670] -> w365
        tunnel: [w669] -> w364
        tunnel: w361 -> [w668]
        tunnel: [w668] -> w359
        tunnel: w349 -> [w667]
        tunnel: [w667] -> w345
        tunnel: [w666] -> w344
        tunnel: w348 -> [w666]
        tunnel: w347 -> [w665]
        tunnel: [w665] -> w343
        tunnel: w346 -> [w664]
        tunnel: [w664] -> w342
        tunnel: [w663] -> w339
        tunnel: w341 -> [w663]
        tunnel: [w662] -> w338
        tunnel: [w661] -> w337
        tunnel: w319 -> [w660]
        tunnel: w317 -> [w659]
        frame #0 {
          n92 = call <vilib>:"IMAQdx Configure Grab.vi"("error in"=w633, "Session In"=w636) -> ("error out"=w634:errorcluster, "Session Out"=w635:T3)  [unwired: 8 in]
          n93 = call <vilib>:"IMAQdx Start Acquisition.vi"("error in"=w657, "Session In"=w658) -> ("error out"=w655:errorcluster, "Session Out"=w656:T3)  [unwired: 8 in]
          n94 = call <vilib>:"IMAQdx Configure Grab.vi"("error in"=w641, "Session In"=w642) -> ("error out"=w638:errorcluster, "Session Out"=w639:T3)  [unwired: 8 in]
          n95 = call <vilib>:"DAQmx Start Task.vi"("task/channels in"=w652, "error in"=w651) -> ("task out"=w650:refnum<k21>, "error out"=w649:errorcluster)  [unwired: 12 in]
        }
        frame #1 {
          n96 = Tick Count (ms)() -> (millisecond timer value=w683:u32)
          n97 = call <vilib>:"DAQmx Start Task.vi"("task/channels in"=w659, "error in"=w660) -> ("task out"=w662:refnum<k21>, "error out"=w661:errorcluster)  [unwired: 12 in]
          n98 = Tick Count (ms)() -> (millisecond timer value=w678:u32)
          n99 = Tick Count (ms)() -> (millisecond timer value=w676:u32)
          n100 = Tick Count (ms)() -> (millisecond timer value=w669:u32)
          n101 = Tick Count (ms)() -> (millisecond timer value=w670:u32)
          n102 = call <vilib>:"DAQmx Start Task.vi"("task/channels in"=w684, "error in"=w686) -> ("task out"=w688:refnum<k21>, "error out"=w687:errorcluster)  [unwired: 12 in]
          n103 = To Long Integer(number=w675) -> (32bit integer=w674:i32)
        }
      }
      n104 = while {
        tunnel: w338 -> [w559]
        tunnel: [w557] -> w333
        tunnel: w337 -> [w557]
        tunnel: [w559] -> w334
        stop <- w558 stop-if-true
        n105 = local read "Analog Data"() -> (w558:bool)
      }
      n106 = while {
        tunnel: [w741] -> w511
        tunnel: [w724] -> w502
        tunnel: [w749] -> w474
        tunnel: w476 -> [w748]
        tunnel: w477 -> [w747]
        tunnel: w478 -> [w746]
        tunnel: w479 -> [w718]
        shift-right: [w697] -> _
        shift-left: _ -> [w745]
        shift-right: [w744] -> _
        shift-left: u32 0 ("New Lost") -> [w740]
        shift-right: [w743] -> w517
        shift-left: u32[] [] ("NewBuffNum") -> [w733]
        shift-right: [w742] -> w492
        shift-left: u32[] [] ("NewNumLost") -> [w734]
        tunnel: w384 -> [w738]
        tunnel: w468 -> [w728]
        tunnel: w424 -> [w726]
        tunnel: [w724] -> w430
        tunnel: w405 -> [w723]
        tunnel: w428 -> [w721]
        tunnel: w427 -> [w720]
        tunnel: [w721] -> w331
        tunnel: [w720] -> w332
        tunnel: w345 -> [w703]
        tunnel: w344 -> [w702]
        tunnel: w343 -> [w701]
        tunnel: w342 -> [w700]
        tunnel: w339 -> [w698]
        i -> [w716]
        stop <- w735 stop-if-true
        n107 = Greater?(x=w716, y=w723) -> (0:→"Whisk Cam":bool)
        n108 = call <vilib>:"IMAQdx Get Image.vi"("Buffer Number Mode (Next)"=IMAQdx_Buffer_Number_Mode."Buffer Number", "error in"=w747, "Buffer Number In"=w716, "Image In"=w746, "Session In"=w748) -> ("error out"=w755:errorcluster, "Buffer Number Out"=w697:u32, "Image Out"=w717:T1, "Session Out"=w741:T3)  [unwired: 3 in]
        "Last Whisk Buffer" <- w697
        "?" <- w717
        n109 = Multiply(x=w698, y=w697) -> (x*y=w699:dbl)
        n110 = Round Toward -Infinity(1:w699) -> (0:w696:dbl)
        n111 = Tick Count (ms)() -> (millisecond timer value=w729:u32)
        n112 = Index Array(array=w703, index (row)=w696) -> (element=w709:bool[])  [unwired: 1 in]
        n113 = Index Array(array=w702, index (row)=w696) -> (element=w707:bool[])  [unwired: 1 in]
        n114 = Index Array(array=w701, index (row)=w696) -> (element=w705:bool[])  [unwired: 1 in]
        n115 = Index Array(array=w700, index (row)=w696) -> ()  [unwired: 1 in, 1 out]
        n116 = Subtract(x=w729, y=w728) -> (x-y=w732:u32)
        n117 = Add(x=w697, y=w740) -> (x+y=w739:u32)
        n118 = call "IMAQ ImageToArray"("error in (no error)"=w755, "Image"=w717) -> ("error out"=w754:errorcluster, "Image Pixels (U8)"=w753:u8[][])  [unwired: 2 in, 3 out]
        n119 = Multiply(x=w732, y=1.667e-05) -> (x*y=w731:dbl)
        n120 = call <vilib>:"Calculate Frames per Second.vi"("Update Interval (ms)"=u32 2000, "Buffer Number"=w697) -> ("Processed Frames/s"=→"Whisk Cam Fs":dbl)  [unwired: 7 in, 2 out]
        n121 = call "TrackDroppedFrames_2P.vi"("NumLost"=w734, "BuffNum"=w733, "Curr Buffer"=w697, "Prev Lost"=w740, "Prev Buffer"=w745) -> ("New Lost"=w744:u32, "NewNumLost"=w742:u32[], "NewBuffNum"=w743:u32[])  [unwired: 4 in]
        "Dropped" <- w744
        n122 = Greater?(x=w709, y=FALSE ("Boolean")) -> (0:w708:bool[])
        n123 = Greater?(x=w707, y=FALSE ("Boolean")) -> (0:w706:bool[])
        n124 = Greater?(x=w705, y=FALSE ("Boolean")) -> (0:w704:bool[])
        n125 = Greater Or Equal?(x=w739, y=w738) -> (x >= y?=w736:bool)
        n126 = Bundle("Time (min)"=w726, w731) -> (→"Time Elapsed (Min)":cluster{"Time (min)":dbl, dbl})  [unwired: 1 in]
        n127 = Write to Binary File(file (use dialog)=w718, data=w753, error in=w754, 5:FALSE ("prepend array or string size? (T)"), 9:T8."little-endian" ("byte order (0:big-endian, network order)")) -> (refnum out=w749:refnum<file>, error out=w724:errorcluster)  [unwired: 1 in, 1 out]
        n128 = Or Array Elements(Boolean array=w708) -> (logical OR=→"LPad":bool)
        n129 = Or Array Elements(Boolean array=w706) -> (logical OR=→"Auditory":bool)
        n130 = Or Array Elements(Boolean array=w704) -> (logical OR=→"RPad":bool)
        n131 = Unbundle By Name(w724) -> ("status"=w737:bool)
        n132 = Compound Arithmetic op=OR(w737, w736, "stop") -> (w735:bool)
        "Whisker Camera" <- w735
      }
      n133 = while {
        tunnel: w487 -> [w623]
        tunnel: w488 -> [w622]
        tunnel: w489 -> [w621]
        tunnel: [w620] -> w509
        tunnel: [w608] -> w325
        tunnel: [w619] -> w326
        shift-right: [w612] -> _
        shift-left: w405 -> [w613]
        tunnel: w405 -> [w604]
        tunnel: w383 -> [w602]
        i -> [w605]
        stop <- w609 stop-if-true
        n134 = Greater?(x=w605, y=w604) -> (0:→"Analog":bool)
        n135 = call-poly <vilib>:"DAQmx Read.vi"("task/channels in"=w622, "error in"=w623) -> ("task out"=w619:refnum<k21>, "data"=w617:waveform(dbl)[], "error out"=w611:errorcluster)  [unwired: 11 in]
        n136 = Index Array(array=w617, index=0) -> (element=w615:waveform(dbl))
        n137 = Unbundle By Name(w615) -> ("Y"=w614:dbl[])
        n138 = Array Size(array=w614) -> (size(s)=w607:i32)
        n139 = TDMS Write(0:w621, 5:"Analog Data" ("group name in (Untitled)"), 9:w617, 11:w611) -> (4:w620:refnum<k34>, 15:w608:errorcluster)  [unwired: 2 in, 2 out]
        n140 = Add(x=w607, y=w613) -> (x+y=w612:u32)
        "Analog Samples" <- w612
        n141 = local read "stop"() -> (w603:bool)
        n142 = Greater Or Equal?(x=w612, y=w602) -> (x >= y?=w610:bool)
        n143 = Compound Arithmetic op=OR(w603, w608, w610) -> (w609:bool)
        "Analog Data" <- w609
      }
      n144 = while {
        tunnel: w404 -> [w588]
        tunnel: w402 -> [w587]
        tunnel: w403 -> [w591]
        tunnel: w399 -> [w590]
        tunnel: [w581] -> w406
        tunnel: [w592] -> w409
        tunnel: [w590] -> w410
        tunnel: w397 -> [w594]
        tunnel: w396 -> [w593]
        i -> [w595]
        stop <- w583 stop-if-true
        n145 = Tick Count (ms)() -> (millisecond timer value=w599:u32)
        n146 = Greater?(x=w594, y=w595) -> (0:→"Behav Cam":bool)
        n147 = Subtract(x=w599, y=w593) -> (x-y=w600:u32)
        n148 = Divide(x=w600, y=u32 1000) -> (x/y=w589:dbl)
        n149 = call "GrabWebCam_2P.vi"("Session In"=w587, "Image In"=w588, "Trial Time"=w589, "AVI Refnum"=w590, "error in"=w591) -> ("Session Out"=w581:T3, "WebCam Img Out"=→"?":T1, "Buffer Number Out"=w585:u32, "error out"=w592:errorcluster)  [unwired: 7 in]
        n150 = call <vilib>:"Calculate Frames per Second.vi"("Update Interval (ms)"=u32 5000, "Buffer Number"=w585) -> ("Processed Frames/s"=→"Web Cam Fs":dbl)  [unwired: 7 in, 2 out]
        n151 = local read "Analog Data"() -> (w584:bool)
        n152 = local read "stop"() -> (w582:bool)
        n153 = Compound Arithmetic op=OR(w582, w584) -> (w583:bool)
      }
      n154 = while {
        tunnel: [w566] -> w356
        tunnel: [w573] -> w355
        tunnel: w365 -> [w565]
        tunnel: w364 -> [w564]
        tunnel: w363 -> [w563]
        tunnel: w362 -> [w562]
        tunnel: w359 -> [w561]
        tunnel: [w560] -> w354
        tunnel: w353 -> [w560]
        i -> [w574]
        stop <- w568 stop-if-true
        n155 = Tick Count (ms)() -> (millisecond timer value=w578:u32)
        n156 = Greater?(x=w564, y=w574) -> (0:→"MScan Cam":bool)
        n157 = Subtract(x=w578, y=w565) -> (x-y=w579:u32)
        n158 = Divide(x=w579, y=u32 1000) -> (x/y=w572:dbl)
        n159 = call "GrabWebCam_2P.vi"("Session In"=w563, "Image In"=w561, "Trial Time"=w572, "AVI Refnum"=w560, "error in"=w562) -> ("Session Out"=w566:T3, "WebCam Img Out"=→"?":T1, "Buffer Number Out"=w570:u32, "error out"=w573:errorcluster)  [unwired: 7 in]
        n160 = call <vilib>:"Calculate Frames per Second.vi"("Update Interval (ms)"=u32 5000, "Buffer Number"=w570) -> ("Processed Frames/s"=→"Web Cam Fs 2":dbl)  [unwired: 7 in, 2 out]
        n161 = local read "Analog Data"() -> (w569:bool)
        n162 = local read "stop"() -> (w567:bool)
        n163 = Compound Arithmetic op=OR(w567, w569) -> (w568:bool)
      }
      n164 = Delete From Array(array=w492, length=1, index=0) -> (array with subset deleted=w523:u32[])  [unwired: 1 out]
      n165 = Delete From Array(array=w517, length=1, index=0) -> (array with subset deleted=w524:u32[])  [unwired: 1 out]
      n166 = Close File(refnum=w474, error in=w502) -> (path=w494:path, error out=w495:errorcluster)
      n167 = call <vilib>:"IMAQdx Close Camera.vi"("error in"=w430, "Session In"=w511) -> ()  [unwired: 9 in, 1 out]
      n168 = call <vilib>:"IMAQdx Close Camera.vi"("error in"=w409, "Session In"=w406) -> ()  [unwired: 9 in, 1 out]
      n169 = call "IMAQ AVI2 Close"("error in (no error)"=w409, "AVI Refnum"=w410) -> ("error out"=w408:errorcluster)  [unwired: 9 in]
      n170 = call <vilib>:"IMAQdx Close Camera.vi"("error in"=w355, "Session In"=w356) -> ()  [unwired: 9 in, 1 out]
      n171 = call "IMAQ AVI2 Close"("error in (no error)"=w355, "AVI Refnum"=w354) -> ("error out"=w358:errorcluster)  [unwired: 9 in]
      n172 = Move(source path=w494, error in=w495, 10:"Target Path") -> (error out=w497:errorcluster)  [unwired: 2 in, 2 out]
      n173 = Build Array(w524, w523) -> (w521:u32[][])
      n174 = Move(source path=w352, error in=w408, 10:"Target Path") -> (error out=w407:errorcluster)  [unwired: 2 in, 2 out]
      n175 = Move(source path=w350, error in=w358, 10:"Target Path") -> (error out=w357:errorcluster)  [unwired: 2 in, 2 out]
      n176 = flat-sequence {
        tunnel: [w550] -> w336
        tunnel: [w549] -> w335
        tunnel: w334 -> [w539]
        tunnel: w333 -> [w548]
        tunnel: w332 -> [w547]
        tunnel: w331 -> [w546]
        tunnel: [w545] -> w330
        tunnel: [w544] -> w329
        tunnel: [w543] -> w328
        tunnel: [w542] -> w327
        tunnel: w326 -> [w541]
        tunnel: w325 -> [w540]
        tunnel: w336 -> [w556]
        tunnel: w335 -> [w555]
        tunnel: w330 -> [w554]
        tunnel: w329 -> [w553]
        tunnel: w328 -> [w552]
        tunnel: w327 -> [w551]
        frame #0 {
          n177 = call <vilib>:"DAQmx Stop Task.vi"("task/channels in"=w541, "error in"=w540) -> ("task out"=w543:refnum<k21>, "error out"=w542:errorcluster)  [unwired: 12 in]
          n178 = call <vilib>:"DAQmx Stop Task.vi"("task/channels in"=w547, "error in"=w546) -> ("task out"=w544:refnum<k21>, "error out"=w545:errorcluster)  [unwired: 12 in]
          n179 = call <vilib>:"DAQmx Stop Task.vi"("task/channels in"=w539, "error in"=w548) -> ("task out"=w550:refnum<k21>, "error out"=w549:errorcluster)  [unwired: 12 in]
        }
        frame #1 {
          n180 = call <vilib>:"DAQmx Clear Task.vi"("task in"=w552, "error in"=w551) -> ()  [unwired: 13 in, 1 out]
          n181 = call <vilib>:"DAQmx Clear Task.vi"("task in"=w553, "error in"=w554) -> ()  [unwired: 13 in, 1 out]
          n182 = call <vilib>:"DAQmx Clear Task.vi"("task in"=w556, "error in"=w555) -> ()  [unwired: 13 in, 1 out]
        }
      }
      n183 = Array To Spreadsheet String(delimiter (Tab)=",", array=w524, 3:"%d" ("format string")) -> (spreadsheet string=w513:string)
      n184 = Array To Spreadsheet String(delimiter (Tab)=",", array=w523, 3:"%d" ("format string")) -> (spreadsheet string=w514:string)
      n185 = Transpose 2D Array(2D array=w521) -> (transposed array=w522:u32[][])
      n186 = call <vilib>:"Simple Error Handler.vi"("error in (no error)"=w497) -> ()  [unwired: 1 in, 8 out]
      n187 = call <vilib>:"Trim Whitespace.vi"("string"=w513) -> ("trimmed string"=w382:string)  [unwired: 1 in]
      n188 = call <vilib>:"Trim Whitespace.vi"("string"=w514) -> ("trimmed string"=w515:string)  [unwired: 1 in]
      n189 = call <vilib>:"Simple Error Handler.vi"("error in (no error)"=w407) -> ()  [unwired: 1 in, 8 out]
      n190 = call <vilib>:"Simple Error Handler.vi"("error in (no error)"=w357) -> ()  [unwired: 1 in, 8 out]
      n191 = Number To Decimal String(number=w522) -> ()  [unwired: 1 in, 1 out]
      n192 = Build Array(w382, w515) -> (w516:string[])
      n193 = TDMS Set Properties(5:w516, 7:string[] ["WhiskerCam_DroppedFrameIndex", "WhiskerCam_NumberDropped"] ("channel name(s) in (Untitled)"), 8:w325, 11:w509) -> (0:w510:errorcluster, 3:w512:refnum<k34>)  [unwired: 2 in, 2 out]
      n194 = TDMS Close(8:w510, 11:w512) -> (0:w493:errorcluster, 3:w498:path)
      n195 = Path To String(path=w498) -> (string=w381:string)
      n196 = Concatenate Strings(w381, "_index" ("string")) -> (w499:string)
      n197 = TDMS Defragment(4:w493, 7:w498) -> (0:w501:errorcluster)
      n198 = String To Path(string=w499) -> (path=w500:path)
      n199 = Move(source path=w498, error in=w501, 10:"Target Path") -> (error out=w496:errorcluster)  [unwired: 2 in, 2 out]
      n200 = Move(source path=w500, error in=w501, 10:"Target Path") -> (error out=w380:errorcluster)  [unwired: 2 in, 2 out]
      n201 = call <vilib>:"Simple Error Handler.vi"("error in (no error)"=w380) -> ()  [unwired: 1 in, 8 out]
      n202 = call <vilib>:"Simple Error Handler.vi"("error in (no error)"=w496) -> ()  [unwired: 1 in, 8 out]
    }
    frame #4 {
      "Complete" <- TRUE ("Data Acquisition - Complete")
    }
  }
